vi "LVClass_ModalCoef GetCoefValues.vi"(0 "ModalCoef in":refnum<class "ModalCoef.lvclass">, 11 "error in (no error)":errorcluster) -> (4 "ModalCoef out":refnum<class "ModalCoef.lvclass">, 6 "coef":sgl[](array[numeric]), 8 "index":u32[](array[numeric]), 15 "error out":errorcluster)   [LabVIEW 2020, in "ModalCoef.lvclass"]
doc: "Get polynomial coefficients informations and values.\n\n--------------------------------------------------------------------------------\n\n<B>TypePhaseIn </B> : TypePhase phase mode reconstruction.\n<B>TypePhaseOut </B> : TypePhase phase mode reconstruction.\n<B>modalCoef </B> : ModalCoef object.\n<B>coef </B> : Array of modal coefficient values.\n<B>index </B> : Array of modal coefficient indices.\n<B>pupil </B> : pupil object.\n<B>ErrorIn </B> : Error\n<B>ErrorOut </B> : Error\n\n--------------------------------------------------------------------------------"
uses:
  ModalCoef.lvclass
  ModalCoef.lvclass/ModalCoef.ctl
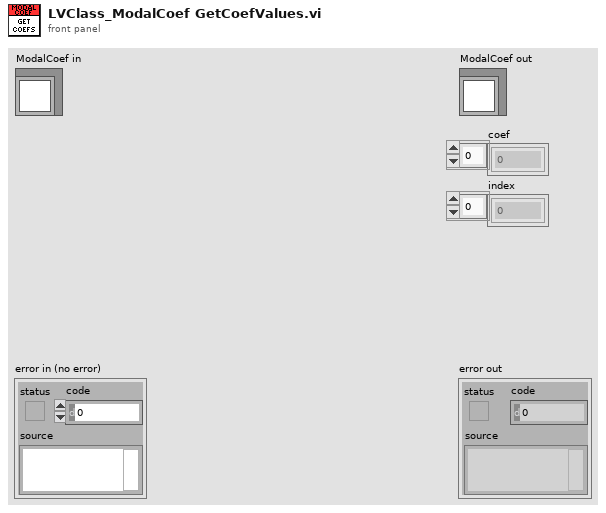
[diagram p1: front panel]
types:
  T1 = typedef "ClassID.ctl" = i64
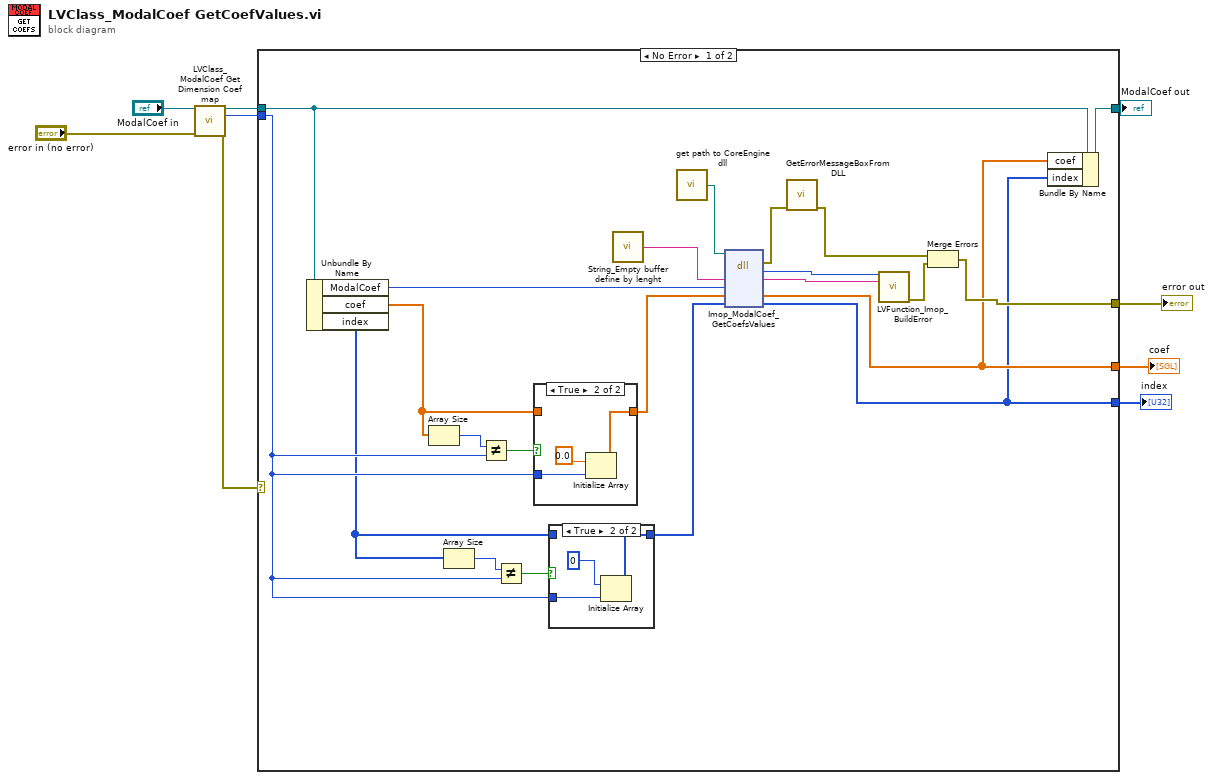
[diagram p0: block diagram]
diagram:
  n1 = call "LVClass_ModalCoef Get Dimension Coef map.vi"("ModalCoef in"="ModalCoef in", "error in (no error)"="error in (no error)") -> ("ModalCoef out"=w4:refnum<class "ModalCoef.lvclass">, "# of coef"=w1:i32, "error out"=w2:errorcluster)  [unwired: 11 in]
  n2 = case shown="No Error" w2 {
    selector: w2 -> [_ w41]
    tunnel: [w23 w41] -> w9
    tunnel: [w12 w40] -> w8
    tunnel: w4 -> [w13 w40]
    tunnel: [w11 _] -> w7
    tunnel: [w10 _] -> w6
    tunnel: w1 -> [w16 _]
    frame No Error {
      n3 = Unbundle By Name(w13) -> ("ModalCoef"=w31:T1, "coef"=w22:sgl[], "index"=w15:u32[])
      n4 = Array Size(array=w22) -> (size(s)=w21:i32)
      n5 = Array Size(array=w15) -> (size(s)=w17:i32)
      n6 = Not Equal?(x=w21, y=w16) -> (x != y?=w20:bool)
      n7 = Not Equal?(x=w17, y=w16) -> (x != y?=w18:bool)
      n8 = case shown="True" w20 {
        tunnel: [w36 w38] -> w19
        tunnel: w16 -> [_ w39]
        tunnel: w22 -> [w36 _]
        frame False {
        }
        frame True {
          n9 = Initialize Array(sgl 0.0, w39) -> (w38:sgl[])
        }
      }
      n10 = case shown="True" w18 {
        tunnel: [w32 w34] -> w14
        tunnel: w16 -> [_ w35]
        tunnel: w15 -> [w32 _]
        frame False {
        }
        frame True {
          n11 = Initialize Array(u32 0, w35) -> (w34:u32[])
        }
      }
      n12 = call "String_Empty buffer define by lenght.vi"() -> ("Empty buffer"=w30:string)  [unwired: 1 in]
      n13 = call "get path to CoreEngine dll.vi"() -> ("path to wavekit library"=w27:path)  [unwired: 14 in, 1 out]
      n14 = dll-call lib="D:/2_trunk/Soft_haso/ImOpCoreEngine4_LV2011/DLLs/ImopEngine4_vc100.dll" fn="Imop_ModalCoef_GetCoefsValues"(path in=w27, "message"=w30, "ModalCoef"=w31, "coef"=w19, "index"=w14) -> (error out=w26:errorcluster, "return type"=w28:i32, "message"=w29:string, "coef"=w11:sgl[], "index"=w10:u32[])  [unwired: 3 in, 1 out]
      n15 = call "GetErrorMessageBoxFromDLL.vi"("error IN"=w26) -> ("error OUT"=w25:errorcluster)  [unwired: 10 in]
      n16 = call "LVFunction_Imop_BuildError.vi"("code"=w28, "String to Prepend to source (\"\")"=w29) -> ("error out"=w24:errorcluster)  [unwired: 13 in]
      n17 = Merge Errors(w25, w24) -> (w23:errorcluster)
      n18 = Bundle By Name(cluster=w13, "coef"=w11, "index"=w10) -> (w12:refnum<class "ModalCoef.lvclass">)
    }
    frame Error {
    }
  }
  "error out" <- w9
  "ModalCoef out" <- w8
  "index" <- w6
  "coef" <- w7
